vi "DeCRC.vi"(6 "F":dbl, 8 "error in (no error)":errorcluster caption="错误输入（无错误）", 9 "deldpccode":dbl[][](array[numeric]), 10 "C":dbl, 11 "appended path":path) -> (0 "error IO":errorcluster, 3 "tbdata":dbl[](array[numeric]), 4 "crcflag":dbl)   [LabVIEW 2015]
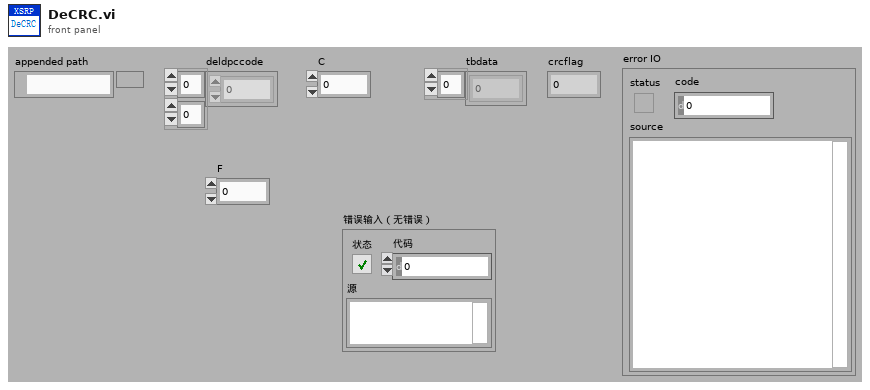
[diagram p1: front panel]
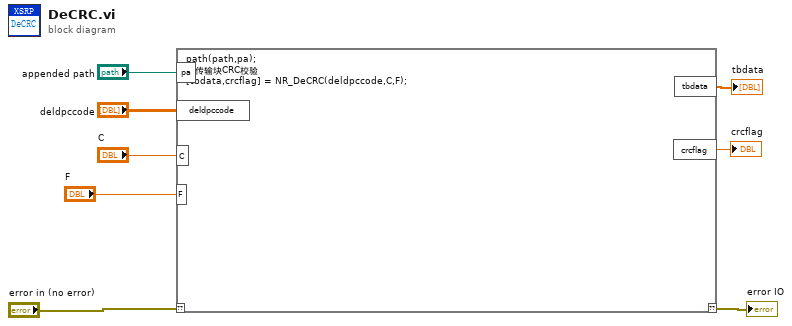
[diagram p0: block diagram]
diagram:
  n1 = script code="path(path,pa);\n%传输块CRC校验\n[tbdata,crcflag] = NR_DeCRC(deldpccode,C,F);"("??"="error in (no error)", "pa"="appended path", "deldpccode"="deldpccode", "C"="C", "F"="F") -> ("??"=→"error IO":errorcluster, "tbdata"=→"tbdata":dbl[], "crcflag"=→"crcflag":dbl)
